vi "LDA_IP.vi"() -> (0 "error out":errorcluster)   [LabVIEW 2017]
uses:
  Globals/Meas_global.vi
  Globals/LDA_meas_global_2.vi
  Globals/LDA_meas_global_1.vi
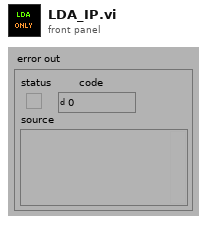
[diagram p1: front panel]
types:
  T1 = typedef "Analysis_info_cluster.ctl" = cluster{"Colour":u32, "Inst type":T2, "Inst name":string, "Symbol":string, "Code name":string, "Extra Info":string, "Inst Array":T3, "Extra Titles":string[], "Extra Values":string[], "U":dbl, "u^2":dbl, "u^3":dbl, "u^4":dbl, "Skew_u":dbl, "Kurt_u":dbl, "Sd Error in Mean":dbl, "% u'/U":dbl, "X":dbl, "Y":dbl, "Z":dbl, "Timescale integral Estimate":dbl, "Sd Error in Variance":dbl, "Calib File":path, "Calib Constants":dbl[], "Output Position":bool, "Full Stats":bool, "Av Sampling Rate":dbl, "Av No of Samples":dbl, "Total Meas Time (s)":dbl, "ADAM Ch Name":string, "Max value":dbl, "Min value":dbl, "Req Sample Rate Hz":dbl, "Sync Delay Time (s)":dbl, "Ch No":i16, "Device ID":string, "Use Latest Calib":bool}
  T2 = typedef "Inst_type.ctl" = enum16{"Propeller anemometer", "Raw voltage", "Pressure Transducer", "Pitot-static tube", "Preston tube", "Hot wire", "Cross wire 1", "Cross wire 2", "Generic Linear", "Generic Polynomial", "Generic BackPoly", "Fast FID", "Thermocouple", "Cold wire", "Pulsed Wire", "LDA Vel", "LDA Tran time", "LDA Arr time", "Microphone"}
  T3 = typedef "Instrument_Array.ctl" = enum16{"PWA", "LDA", "Analogue"}
  T4 = typedef "LDA_Setup.ctl" = cluster{"dimensions":enum16{"1D", "2D"}, "Analogue Freq Multiplier":dbl}
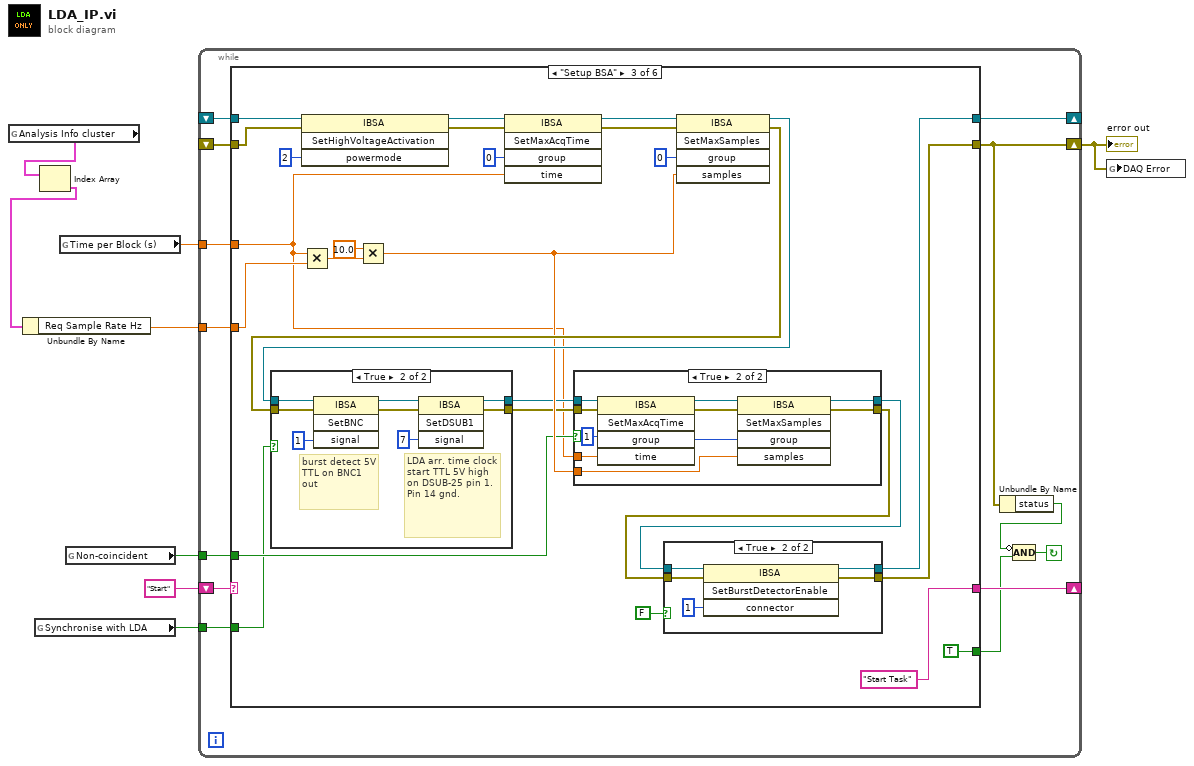
[diagram p0: block diagram]
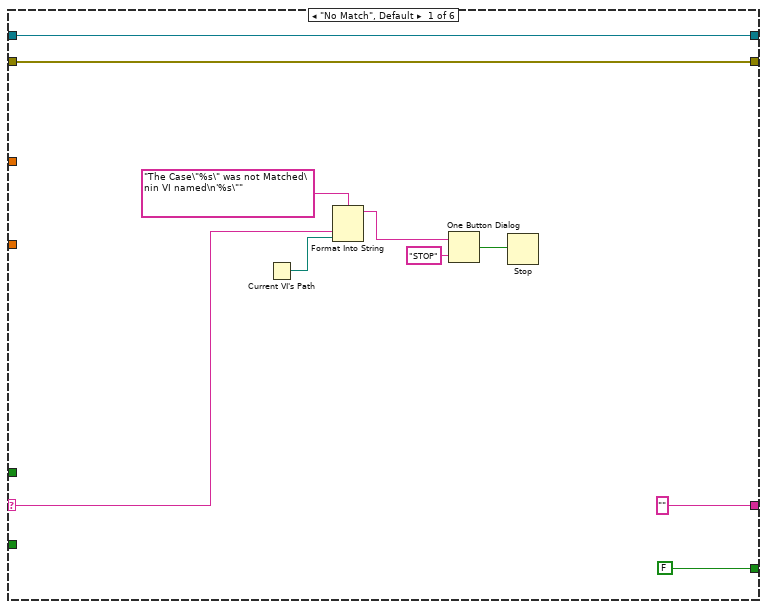
[diagram p2: hidden frame]
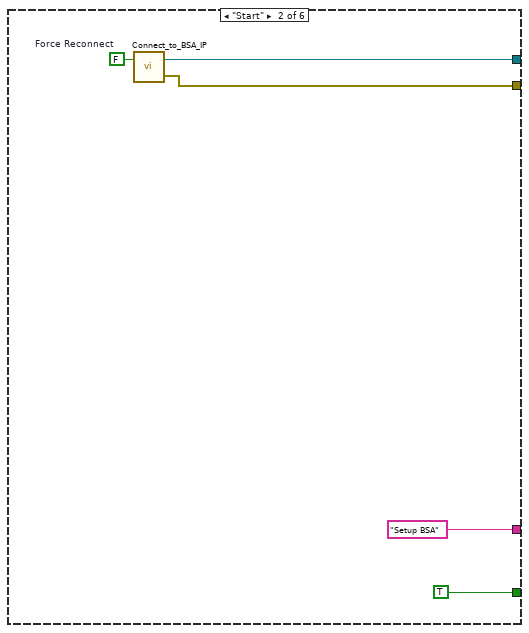
[diagram p3: hidden frame]
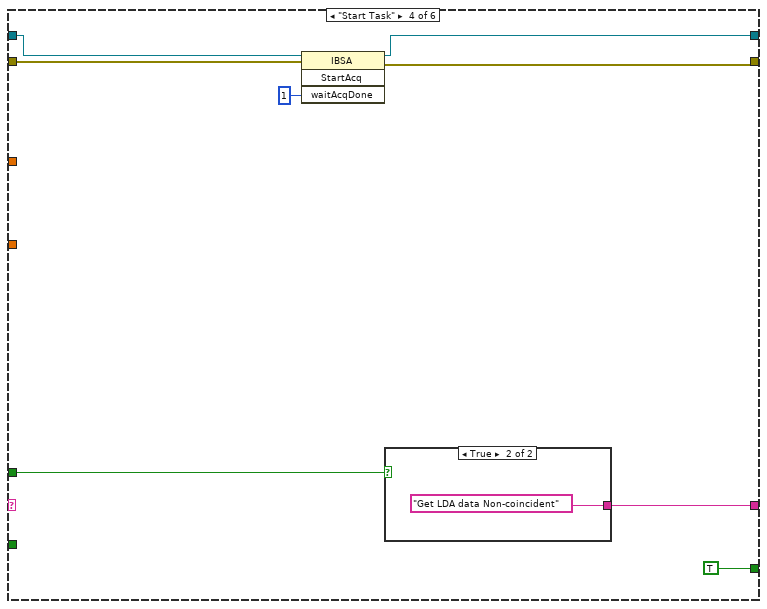
[diagram p7: hidden frame]
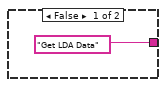
[diagram p8: hidden frame]
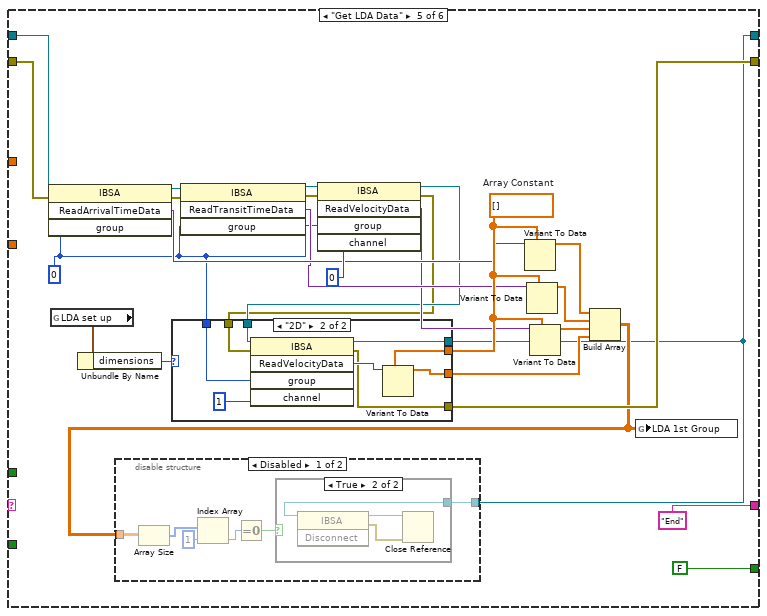
[diagram p9: hidden frame]
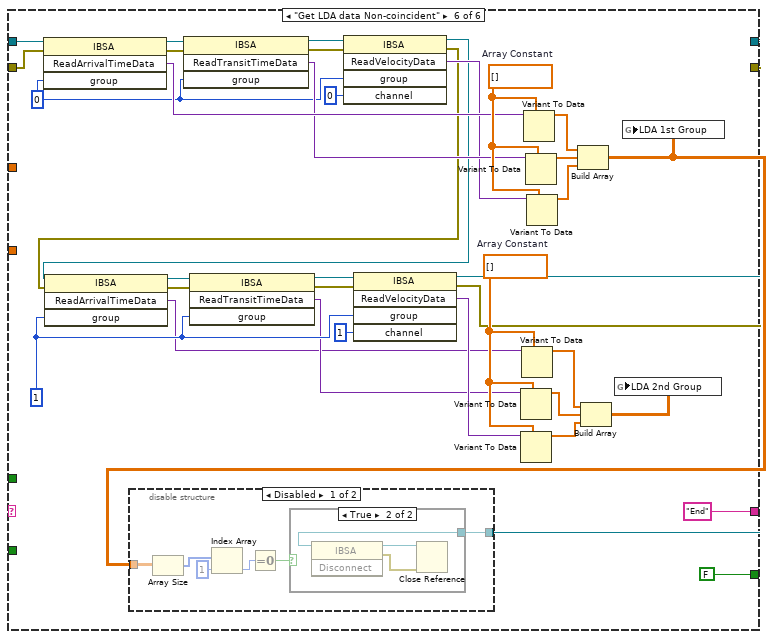
[diagram p13: hidden frame]
diagram:
  n1 = global read "Meas_global.vi" "Analysis Info cluster"() -> (w4:T1[])
  n2 = global read "Meas_global.vi" "Synchronise with LDA"() -> (w7:bool)
  n3 = Index Array(array=w4) -> (element=w3:T1)  [unwired: 1 in]
  n4 = Unbundle By Name(w3) -> ("Req Sample Rate Hz"=w2:dbl)
  n5 = global read "Meas_global.vi" "Time per Block (s)"() -> (w1:dbl)
  n6 = global read "LDA_meas_global_1.vi" "Non-coincident"() -> (w6:bool)
  n7 = while {
    shift-left: "Start" -> [w20]
    shift-right: [w21] -> _
    shift-right: [w13] -> w5
    shift-left: _ -> [w19]
    tunnel: w2 -> [w18]
    shift-right: [w16] -> _
    shift-left: _ -> [w17]
    tunnel: w7 -> [w15]
    tunnel: w6 -> [w14]
    tunnel: w1 -> [w9]
    stop <- w11 continue-if-true
    n8 = case shown="\"Setup BSA\"" w20 {
      selector: w20 -> [w22 _ _ _ _ _]
      tunnel: [FALSE TRUE TRUE TRUE FALSE FALSE] -> w10
      tunnel: ["" "Setup BSA" "Start Task" w94 "End" "End"] -> w21
      tunnel: [w24 w34 w41 w98 w109 w157] -> w13
      tunnel: w19 -> [w24 _ w55 w95 w107 w155]
      tunnel: w18 -> [_ _ w47 _ _ _]
      tunnel: w17 -> [w23 _ w56 w97 w113 w156]
      tunnel: [w23 w35 w42 w96 w104 w149] -> w16
      tunnel: w15 -> [_ _ w40 _ _ _]
      tunnel: w14 -> [_ _ w49 w93 _ _]
      tunnel: w9 -> [_ _ w37 _ _ _]
      frame "No Match", Default {
        n9 = Current VI's Path() -> (path=w26:path)
        n10 = Format Into String(format string="The Case\"%s\" was not Matched\nin VI named\n'%s\"" ("Format String"), w22, w26) -> (resulting string=w29:string)  [unwired: 2 in, 1 out]
        n11 = One Button Dialog(message=w29, button name ("OK")="STOP") -> (true=w27:bool)
        n12 = Stop(stop? (T)=w27) -> ()
      }
      frame "Start" {
        w32 = FALSE  # Force Reconnect
        n13 = call "Connect_to_BSA_IP.vi"("Force Reconnect"=w32) -> ("error out"=w34:errorcluster, "BSA"=w35:refnum<k7>)  [unwired: 1 out]
      }
      frame "Setup BSA" {
        n14 = invoke class="IBSA" method="SetHighVoltageActivation"(reference=w56, error in=w55, "powermode"=2) -> (reference out=w61:refnum<k7>, error out=w63:errorcluster)  [unwired: 1 in, 2 out]
        n15 = Multiply(x=w37, y=w47) -> (x*y=w46:dbl)
        n16 = Multiply(x=10.0 ("y"), y=w46) -> (x*y=w50:dbl)
        n17 = invoke class="IBSA" method="SetMaxAcqTime"(reference=w61, error in=w63, "group"=0, "time"=w37) -> (reference out=w62:refnum<k7>, error out=w60:errorcluster)  [unwired: 1 in, 3 out]
        n18 = invoke class="IBSA" method="SetMaxSamples"(reference=w62, error in=w60, "group"=0, "samples"=w50) -> (reference out=w52:refnum<k7>, error out=w51:errorcluster)  [unwired: 1 in, 3 out]
        n19 = case shown="True" w40 {
          tunnel: w52 -> [w82 w90]
          tunnel: w51 -> [w83 w89]
          tunnel: [w82 w86] -> w39
          tunnel: [w83 w85] -> w38
          frame False {
          }
          frame True {
            # "LDA arr. time clock start TTL 5V high on DSUB-25 pin 1. Pin 14 gnd."
            # "burst detect 5V TTL on BNC1 out"
            n20 = invoke class="IBSA" method="SetBNC"(reference=w90, error in=w89, "signal"=1) -> (reference out=w88:refnum<k7>, error out=w87:errorcluster)  [unwired: 1 in, 2 out]
            n21 = invoke class="IBSA" method="SetDSUB1"(reference=w88, error in=w87, "signal"=7) -> (reference out=w86:refnum<k7>, error out=w85:errorcluster)  [unwired: 1 in, 2 out]
          }
        }
        n22 = case shown="True" w49 {
          tunnel: w39 -> [w72 w79]
          tunnel: [w72 w77] -> w44
          tunnel: w38 -> [w71 w76]
          tunnel: [w71 w75] -> w43
          tunnel: w37 -> [_ w74]
          tunnel: w50 -> [_ w73]
          frame False {
          }
          frame True {
            w80 = 1 ("group")
            n23 = invoke class="IBSA" method="SetMaxAcqTime"(reference=w79, error in=w76, "group"=w80, "time"=w74) -> (reference out=w78:refnum<k7>, error out=w81:errorcluster)  [unwired: 1 in, 3 out]
            n24 = invoke class="IBSA" method="SetMaxSamples"(reference=w78, error in=w81, "group"=w80, "samples"=w73) -> (reference out=w77:refnum<k7>, error out=w75:errorcluster)  [unwired: 1 in, 3 out]
          }
        }
        n25 = case shown="True" FALSE {
          tunnel: w44 -> [w65 w70]
          tunnel: w43 -> [w64 w69]
          tunnel: [w65 w68] -> w42
          tunnel: [w64 w67] -> w41
          frame False {
          }
          frame True {
            n26 = invoke class="IBSA" method="SetBurstDetectorEnable"(reference=w70, error in=w69, "connector"=1) -> (reference out=w68:refnum<k7>, error out=w67:errorcluster)  [unwired: 1 in, 2 out]
          }
        }
      }
      frame "Start Task" {
        n27 = invoke class="IBSA" method="StartAcq"(reference=w97, error in=w95, "waitAcqDone"=1) -> (reference out=w96:refnum<k7>, error out=w98:errorcluster)  [unwired: 1 in, 2 out]
        n28 = case shown="True" w93 {
          tunnel: ["Get LDA Data" "Get LDA data Non-coincident"] -> w94
          frame False {
          }
          frame True {
          }
        }
      }
      frame "Get LDA Data" {
        w121 = dbl[] []  # Array Constant
        w110 = 0 ("group")
        n29 = invoke class="IBSA" method="ReadArrivalTimeData"(reference=w113, error in=w107, "group"=w110) -> (reference out=w126:refnum<k7>, error out=w125:errorcluster, "ReadArrivalTimeData"=w120:variant)  [unwired: 1 in, 1 out]
        n30 = global read "Meas_global.vi" "LDA set up"() -> (w106:T4)
        n31 = Unbundle By Name(w106) -> ("dimensions"=w105:enum16{"1D", "2D"})
        n32 = invoke class="IBSA" method="ReadTransitTimeData"(reference=w126, error in=w125, "group"=w110) -> (reference out=w124:refnum<k7>, error out=w123:errorcluster, "ReadTransitTimeData"=w119:variant)  [unwired: 1 in, 1 out]
        n33 = invoke class="IBSA" method="ReadVelocityData"(reference=w124, error in=w123, "group"=w110, "channel"=0) -> (reference out=w112:refnum<k7>, error out=w111:errorcluster, "ReadVelocityData"=w118:variant)  [unwired: 1 in, 2 out]
        n34 = case shown="\"2D\"" w105 {
          tunnel: w121 -> [w137 w146]
          tunnel: [w137 w144] -> w114
          tunnel: [w138 w143] -> w104
          tunnel: w112 -> [w138 w142]
          tunnel: w111 -> [w136 w141]
          tunnel: w110 -> [_ w140]
          tunnel: [w136 w139] -> w109
          frame "1D" {
          }
          frame "2D" {
            n35 = invoke class="IBSA" method="ReadVelocityData"(reference=w142, error in=w141, "group"=w140, "channel"=1) -> (reference out=w143:refnum<k7>, error out=w139:errorcluster, "ReadVelocityData"=w145:variant)  [unwired: 1 in, 2 out]
            n36 = Variant To Data(type=w146, Variant=w145) -> (data=w144:dbl[])  [unwired: 1 in, 1 out]
          }
        }
        n37 = Variant To Data(type=w121, Variant=w120) -> (data=w117:dbl[])  [unwired: 1 in, 1 out]
        n38 = Variant To Data(type=w121, Variant=w119) -> (data=w116:dbl[])  [unwired: 1 in, 1 out]
        n39 = Variant To Data(type=w121, Variant=w118) -> (data=w115:dbl[])  [unwired: 1 in, 1 out]
        n40 = Build Array(w117, w116, w115, w114) -> (w108:dbl[][])
        n41 = disable-structure shown="Disabled" {
          disable-tunnel: w108 -> [w128 _]
          disable-tunnel: w104 -> [w127 _]
          frame Disabled {
            n42 = Array Size(array=w128) -> (size(s)=w132:i32[])
            n43 = Index Array(array=w132, index=1) -> (element=w130:i32)
            n44 = Equal To 0?(x=w130) -> (x = 0?=w129:bool)
            n45 = case shown="True" w129 {
              tunnel: w127 -> [_ w134]
              frame False {
              }
              frame True {
                n46 = invoke class="IBSA" method="Disconnect"(reference=w134) -> (reference out=w135:refnum<k7>, error out=w133:errorcluster)  [unwired: 2 in, 1 out]
                n47 = Close Reference(reference=w135, error in (no error)=w133) -> ()  [unwired: 1 out]
              }
            }
          }
          frame Enabled {
          }
        }
        n48 = global write "LDA_meas_global_2.vi" "LDA 1st Group"(w108) -> ()
      }
      frame "Get LDA data Non-coincident" {
        w164 = dbl[] []  # Array Constant
        w171 = 1 ("group")
        w178 = dbl[] []  # Array Constant
        w172 = 0 ("group")
        n49 = invoke class="IBSA" method="ReadArrivalTimeData"(reference=w156, error in=w155, "group"=w172) -> (reference out=w183:refnum<k7>, error out=w182:errorcluster, "ReadArrivalTimeData"=w177:variant)  [unwired: 1 in, 1 out]
        n50 = invoke class="IBSA" method="ReadTransitTimeData"(reference=w183, error in=w182, "group"=w172) -> (reference out=w181:refnum<k7>, error out=w180:errorcluster, "ReadTransitTimeData"=w176:variant)  [unwired: 1 in, 1 out]
        n51 = invoke class="IBSA" method="ReadVelocityData"(reference=w181, error in=w180, "group"=w172, "channel"=0) -> (reference out=w158:refnum<k7>, error out=w159:errorcluster, "ReadVelocityData"=w175:variant)  [unwired: 1 in, 2 out]
        n52 = invoke class="IBSA" method="ReadArrivalTimeData"(reference=w158, error in=w159, "group"=w171) -> (reference out=w166:refnum<k7>, error out=w167:errorcluster, "ReadArrivalTimeData"=w160:variant)  [unwired: 1 in, 1 out]
        n53 = invoke class="IBSA" method="ReadTransitTimeData"(reference=w166, error in=w167, "group"=w171) -> (reference out=w168:refnum<k7>, error out=w169:errorcluster, "ReadTransitTimeData"=w161:variant)  [unwired: 1 in, 1 out]
        n54 = invoke class="IBSA" method="ReadVelocityData"(reference=w168, error in=w169, "group"=w171, "channel"=1) -> (reference out=w149:refnum<k7>, error out=w157:errorcluster, "ReadVelocityData"=w162:variant)  [unwired: 1 in, 2 out]
        n55 = Variant To Data(type=w164, Variant=w161) -> (data=w163:dbl[])  [unwired: 1 in, 1 out]
        n56 = Variant To Data(type=w164, Variant=w162) -> (data=w152:dbl[])  [unwired: 1 in, 1 out]
        n57 = Variant To Data(type=w164, Variant=w160) -> (data=w165:dbl[])  [unwired: 1 in, 1 out]
        n58 = Variant To Data(type=w178, Variant=w177) -> (data=w174:dbl[])  [unwired: 1 in, 1 out]
        n59 = Variant To Data(type=w178, Variant=w176) -> (data=w173:dbl[])  [unwired: 1 in, 1 out]
        n60 = Variant To Data(type=w178, Variant=w175) -> (data=w153:dbl[])  [unwired: 1 in, 1 out]
        n61 = Build Array(w174, w173, w153) -> (w148:dbl[][])
        n62 = disable-structure shown="Disabled" {
          disable-tunnel: w148 -> [w185 _]
          disable-tunnel: w149 -> [w184 _]
          frame Disabled {
            n63 = Array Size(array=w185) -> (size(s)=w189:i32[])
            n64 = Index Array(array=w189, index=1) -> (element=w187:i32)
            n65 = Equal To 0?(x=w187) -> (x = 0?=w186:bool)
            n66 = case shown="True" w186 {
              tunnel: w184 -> [_ w191]
              frame False {
              }
              frame True {
                n67 = invoke class="IBSA" method="Disconnect"(reference=w191) -> (reference out=w192:refnum<k7>, error out=w190:errorcluster)  [unwired: 2 in, 1 out]
                n68 = Close Reference(reference=w192, error in (no error)=w190) -> ()  [unwired: 1 out]
              }
            }
          }
          frame Enabled {
          }
        }
        n69 = Build Array(w165, w163, w152) -> (w154:dbl[][])
        n70 = global write "LDA_meas_global_2.vi" "LDA 2nd Group"(w154) -> ()
        n71 = global write "LDA_meas_global_2.vi" "LDA 1st Group"(w148) -> ()
      }
    }
    n72 = Unbundle By Name(w13) -> ("status"=w12:bool)
    n73 = Compound Arithmetic op=AND(invert w12, w10) -> (w11:bool)
  }
  "error out" <- w5
  n74 = global write "Meas_global.vi" "DAQ Error"(w5) -> ()
